vi "display_3s_stim_3s_ISI_9s_probes_trigger.vi"() -> ()   [LabVIEW 2019]
uses:
  <vilib>/Analysis/Matrix/Datatypes/RealMatrix.ctl
  <vilib>/Utility/file.llb/Write Delimited Spreadsheet (DBL).vi
  <vilib>/Analysis/Matrix/NI_Matrix.lvlib
panel:
  out "Num trials":u32=204
  out "ISI Time":dbl
  out "Stim TS":dbl
  out "Output":dbl[][](array[numeric])
  out "Output frame":T1
  out "Array temp1":T1
  out "Elapsed Time":dbl
  out "Display":bool=TRUE
  out "Trial":u32=1
  out "reward":dbl[](array[numeric])
  out "stim_id":dbl[](array[numeric])
  out "stim_loaded":dbl
  out "Timings":dbl[](array[numeric])
  out "Stimuli Loaded?":bool
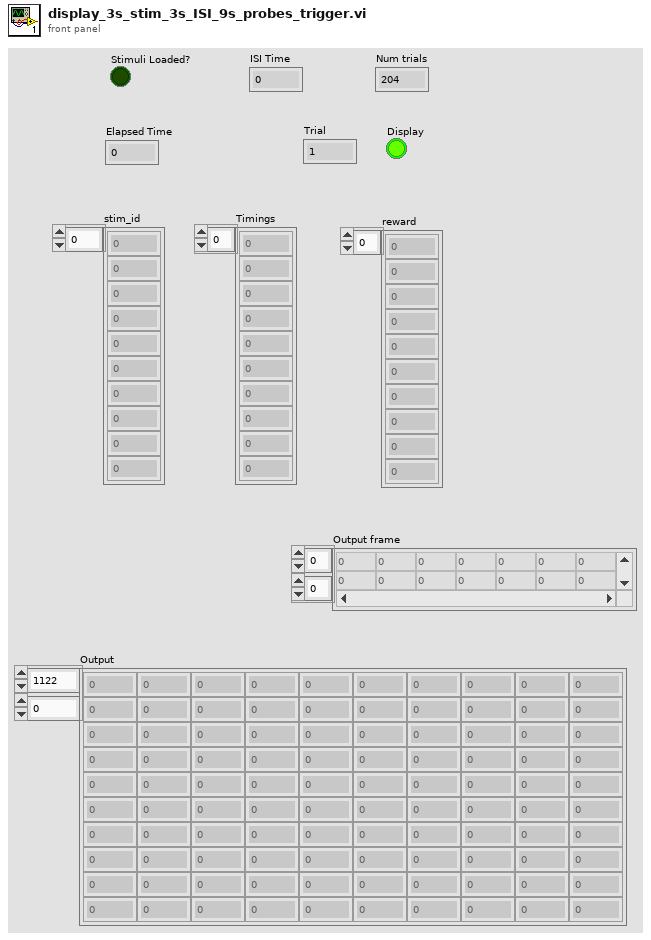
[diagram p1: front panel]
types:
  T1 = typedef "NI_Matrix.lvlib/RealMatrix.ctl" = dbl[][]
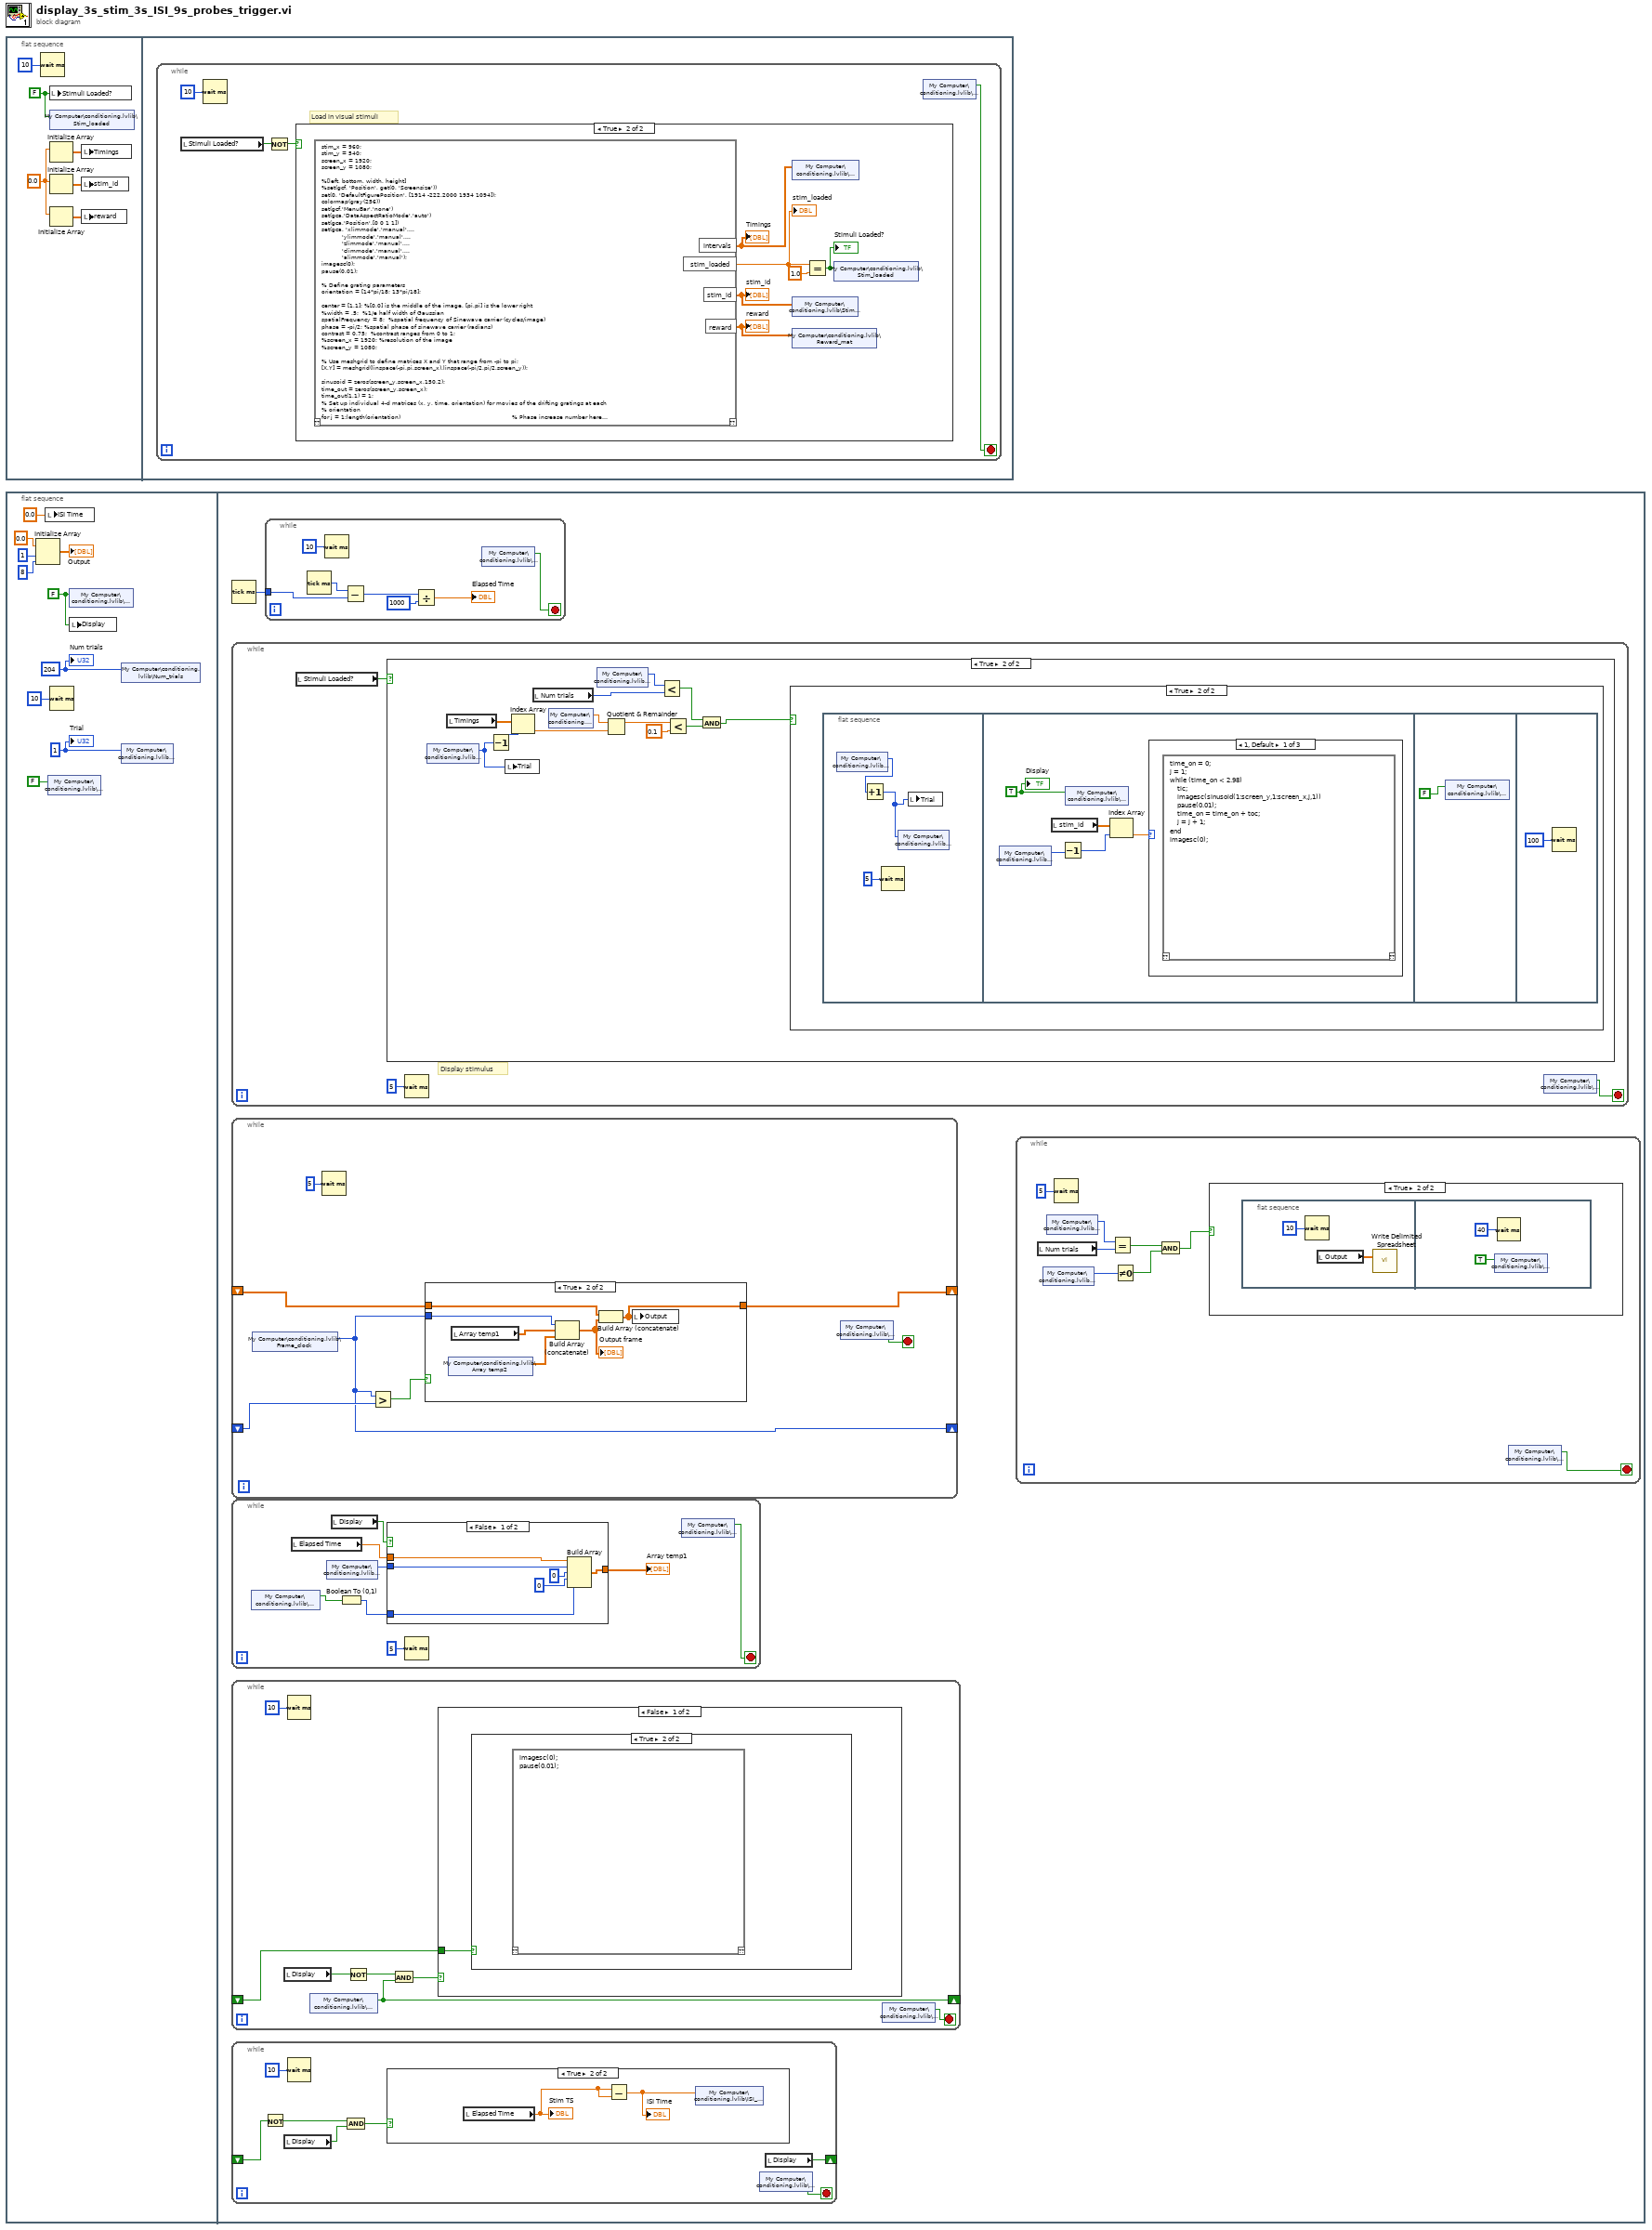
[diagram p0: block diagram]
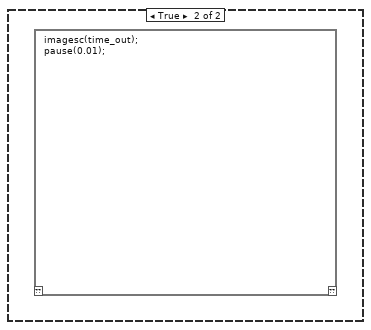
[diagram p5: hidden frame]
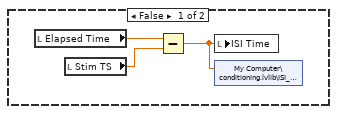
[diagram p6: hidden frame]
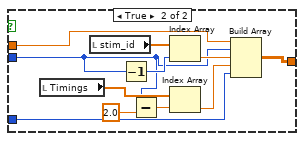
[diagram p7: hidden frame]
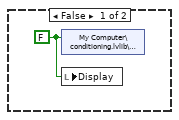
[diagram p10: hidden frame]
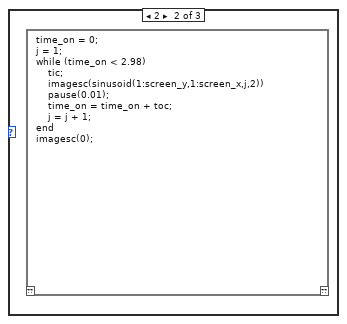
[diagram p11: hidden frame]
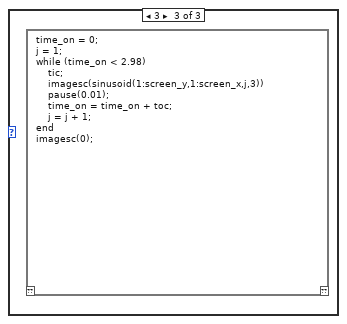
[diagram p12: hidden frame]
diagram:
  n1 = flat-sequence {
    frame #0 {
      w3 = 0.0 ("element")
      w1 = FALSE ("Stimuli Loaded?")
      n2 = Wait (ms)(milliseconds to wait=u32 10) -> ()  [unwired: 1 out]
      n3 = local write "Stimuli Loaded?"(w1) -> ()
      n4 = shared-variable "My Computer\\conditioning.lvlib\\Stim_loaded"(w1) -> ()  [unwired: 1 in, 1 out]
      n5 = Initialize Array(w3) -> (w5:dbl[])  [unwired: 1 in]
      n6 = Initialize Array(w3) -> (w4:dbl[])  [unwired: 1 in]
      n7 = Initialize Array(w3) -> (w2:dbl[])  [unwired: 1 in]
      n8 = local write "Timings"(w5) -> ()
      n9 = local write "stim_id"(w4) -> ()
      n10 = local write "reward"(w2) -> ()
    }
    frame #1 {
      n11 = while {
        stop <- w9 stop-if-true
        # "Load in visual stimuli"
        n12 = local read "Stimuli Loaded?"() -> (w8:bool)
        n13 = Wait (ms)(milliseconds to wait=u32 10) -> ()  [unwired: 1 out]
        n14 = Not(x=w8) -> (.not. x?=w7:bool)
        n15 = case shown="True" w7 {
          frame False {
          }
          frame True {
            n16 = script code="stim_x = 960;\nstim_y = 540;\nscreen_x = 1920;\nscreen_y = 1080;\n\n%[left, bottom, width, height]\n%set(gcf, 'Position', get(0, 'Screensize'))\nset(0, 'DefaultFigurePosition', [1914 -222.2000 1934 1094]);\ncolormap(gray(256))\nset(gcf,'MenuBar','none')\nset(gca,'DataAspectRatioMode','auto')\nset(gca,'Position',[0 0 1 1])\nset(gca, 'xlimmode','manual',...\n           'ylimmode','manual',...\n           'zlimmode','manual',...\n           'climmode','manual',...\n           'alimmode','manual');\nimagesc(0);\npause(0.01);\n\n% Define grating parameters\norientation = [14*pi/18; 13*pi/18];\n\ncenter = [1,1]; %[0,0] is the middle of the image, [pi,pi] is the lower right\n%width = .5;  %1/e half width of Gaussian\nspatialFrequency = 8;  %spatial frequency of Sinewave carrier (cycles/image)\nphase = -pi/2; %spatial phase of sinewave carrier (radians)\ncontrast = 0.75;  %contrast ranges from 0 to 1;\n%screen_x = 1920; %resolution of the image  \n%screen_y = 1080;\n\n% Use meshgrid to define matrices X and Y that range from -pi to pi;\n[X,Y] = meshgrid(linspace(-pi,pi,screen_x),linspace(-pi/2,pi/2,screen_y));\n\nsinusoid = zeros(screen_y,screen_x,150,2);\ntime_out = zeros(screen_y,screen_x);\ntime_out(1,1) = 1;\n% Set up individual 4-d matrices (x, y, time, orientation) for movies of the drifting gratings at each\n% orientation\nfor j = 1:length(orientation)                                                            % Phase increase number here\n    ramp(1:screen_y,1:screen_x,j) = cos(orientation(j))*(X-center(1)) + sin(orientation(j))*(Y-center(2));     %  |\n    for i = 1:150 %Sets the number of frames to define gratings for                   V\n       sinusoid(1:screen_y,1:screen_x,i,j) = contrast*sin(spatialFrequency*ramp(1:screen_y,1:screen_x,j)-...\n           (phase+(2*pi*(i-1)*(-30)/360))); %Number before '/360' sets the phase increase\n    end\nend\n\n%intervals = [ones(1,41)*10 ones(1,41)*11 ones(1,41)*12 ones(1,41)*13 ones(1,40)*14];\nintervals = [];\nfor i = 1:20\n   intervals = [intervals ones(1,9)*3 9];\nend\nintervals = [intervals 3 3 3 3];\n%intervals = [ones(1,204)*3];\nstim_id = [ones(1,204)*1];\n%reward = [ones(1,87)*1 ones(1,15)*0 ones(1,87)*1 ones(1,15)*0];\nreward = [ones(1,204)*1];\n\n%rand_idx1 = randperm(204);\n%rand_idx2 = randperm(204);\n%intervals = intervals(rand_idx2);\n%stim_id = stim_id(rand_idx2);\n%reward = reward(rand_idx2);\n\nstim_loaded = 1;" ("Script Node")() -> ("stim_loaded"=w16:dbl, "intervals"=w11:dbl[], "stim_id"=w12:dbl[], "reward"=w14:dbl[])  [unwired: 1 in, 1 out]
            "stim_loaded" <- w16
            "Timings" <- w11
            "stim_id" <- w12
            "reward" <- w14
            n17 = shared-variable "My Computer\\conditioning.lvlib\\Timings"(w11) -> ()  [unwired: 1 in, 1 out]
            n18 = shared-variable "My Computer\\conditioning.lvlib\\Stim_ID"(w12) -> ()  [unwired: 1 in, 1 out]
            n19 = shared-variable "My Computer\\conditioning.lvlib\\Reward_mat"(w14) -> ()  [unwired: 1 in, 1 out]
            n20 = Equal?(x=w16, y=1.0) -> (x = y?=w13:bool)
            "Stimuli Loaded?" <- w13
            n21 = shared-variable "My Computer\\conditioning.lvlib\\Stim_loaded"(w13) -> ()  [unwired: 1 in, 1 out]
          }
        }
        n22 = shared-variable "My Computer\\conditioning.lvlib\\Stop"() -> (w9:bool)  [unwired: 1 in, 1 out]
      }
    }
  }
  n23 = flat-sequence {
    frame #0 {
      w18 = u32 204
      w24 = FALSE ("Display")
      w26 = u32 1 ("Trial")
      n24 = Initialize Array(0.0 ("element"), 1 ("dimension size"), 8 ("dimension size")) -> (→"Output":dbl[][])
      n25 = local write "ISI Time"(0.0 ("ISI Time")) -> ()
      n26 = shared-variable "My Computer\\conditioning.lvlib\\Stop"(FALSE ("Stop")) -> ()  [unwired: 1 in, 1 out]
      n27 = Wait (ms)(milliseconds to wait=u32 10) -> ()  [unwired: 1 out]
      n28 = shared-variable "My Computer\\conditioning.lvlib\\Display"(w24) -> ()  [unwired: 1 in, 1 out]
      n29 = local write "Display"(w24) -> ()
      n30 = shared-variable "My Computer\\conditioning.lvlib\\Num_trials"(w18) -> ()  [unwired: 1 in, 1 out]
      n31 = shared-variable "My Computer\\conditioning.lvlib\\Trial"(w26) -> ()  [unwired: 1 in, 1 out]
      "Trial" <- w26
      "Num trials" <- w18
    }
    frame #1 {
      n32 = Tick Count (ms)() -> (millisecond timer value=w27:u32)
      n33 = while {
        stop <- w107 stop-if-true
        # "Display stimulus"
        n34 = local read "Stimuli Loaded?"() -> (w106:bool)
        n35 = case shown="True" w106 {
          frame False {
          }
          frame True {
            n36 = shared-variable "My Computer\\conditioning.lvlib\\Trial"() -> (w109:u32)  [unwired: 1 in, 1 out]
            n37 = local read "Timings"() -> (w118:dbl[])
            n38 = Decrement(x=w109) -> (x-1=w111:u32)
            n39 = local write "Trial"(w109) -> ()
            n40 = Index Array(array=w118, index=w111) -> (element=w117:dbl)
            n41 = local read "Num trials"() -> (w114:u32)
            n42 = shared-variable "My Computer\\conditioning.lvlib\\ISI"() -> (w113:dbl)  [unwired: 1 in, 1 out]
            n43 = shared-variable "My Computer\\conditioning.lvlib\\Trial"() -> (w110:u32)  [unwired: 1 in, 1 out]
            n44 = Quotient & Remainder(x=w113, y=w117) -> (x-y*floor(x/y)=w120:dbl)  [unwired: 1 out]
            n45 = Less?(x=w110, y=w114) -> (x < y?=w116:bool)
            n46 = Less?(x=w120, y=0.1) -> (x < y?=w115:bool)
            n47 = And(x=w116, y=w115) -> (x .and. y?=w112:bool)
            n48 = case shown="True" w112 {
              frame False {
                w121 = FALSE ("Display")
                n49 = shared-variable "My Computer\\conditioning.lvlib\\Display"(w121) -> ()  [unwired: 1 in, 1 out]
                n50 = local write "Display"(w121) -> ()
              }
              frame True {
                n51 = flat-sequence {
                  frame #0 {
                    n52 = shared-variable "My Computer\\conditioning.lvlib\\Trial"() -> (w123:u32)  [unwired: 1 in, 1 out]
                    n53 = Increment(x=w123) -> (x+1=w122:u32)
                    n54 = Wait (ms)(milliseconds to wait=u32 5) -> ()  [unwired: 1 out]
                    n55 = shared-variable "My Computer\\conditioning.lvlib\\Trial"(w122) -> ()  [unwired: 1 in, 1 out]
                    n56 = local write "Trial"(w122) -> ()
                  }
                  frame #1 {
                    w128 = TRUE ("Boolean")
                    n57 = shared-variable "My Computer\\conditioning.lvlib\\Trial"() -> (w125:u32)  [unwired: 1 in, 1 out]
                    n58 = local read "stim_id"() -> (w129:dbl[])
                    n59 = Decrement(x=w125) -> (x-1=w126:u32)
                    n60 = shared-variable "My Computer\\conditioning.lvlib\\Display"(w128) -> ()  [unwired: 1 in, 1 out]
                    n61 = Index Array(array=w129, index=w126) -> (element=w127:dbl)
                    n62 = case shown="1, Default" w127 {
                      frame 1, Default {
                        n63 = script code="time_on = 0;\nj = 1;\nwhile (time_on < 2.98)\n    tic;\n    imagesc(sinusoid(1:screen_y,1:screen_x,j,1))\n    pause(0.01);\n    time_on = time_on + toc;\n    j = j + 1;\nend\nimagesc(0);"() -> ()  [unwired: 1 in, 1 out]
                      }
                      frame 2 {
                        n64 = script code="time_on = 0;\nj = 1;\nwhile (time_on < 2.98)\n    tic;\n    imagesc(sinusoid(1:screen_y,1:screen_x,j,2))\n    pause(0.01);\n    time_on = time_on + toc;\n    j = j + 1;\nend\nimagesc(0);"() -> ()  [unwired: 1 in, 1 out]
                      }
                      frame 3 {
                        n65 = script code="time_on = 0;\nj = 1;\nwhile (time_on < 2.98)\n    tic;\n    imagesc(sinusoid(1:screen_y,1:screen_x,j,3))\n    pause(0.01);\n    time_on = time_on + toc;\n    j = j + 1;\nend\nimagesc(0);"() -> ()  [unwired: 1 in, 1 out]
                      }
                    }
                    "Display" <- w128
                  }
                  frame #2 {
                    n66 = shared-variable "My Computer\\conditioning.lvlib\\Display"(FALSE ("Display")) -> ()  [unwired: 1 in, 1 out]
                  }
                  frame #3 {
                    n67 = Wait (ms)(milliseconds to wait=u32 100) -> ()  [unwired: 1 out]
                  }
                }
              }
            }
          }
        }
        n68 = Wait (ms)(milliseconds to wait=u32 5) -> ()  [unwired: 1 out]
        n69 = shared-variable "My Computer\\conditioning.lvlib\\Stop"() -> (w107:bool)  [unwired: 1 in, 1 out]
      }
      n70 = while {
        shift-right: [w96] -> _
        shift-left: _ -> [w97]
        shift-right: [w93] -> _
        shift-left: _ -> [w95]
        stop <- w98 stop-if-true
        n71 = shared-variable "My Computer\\conditioning.lvlib\\Frame_clock"() -> (w93:u32)  [unwired: 1 in, 1 out]
        n72 = Wait (ms)(milliseconds to wait=u32 5) -> ()  [unwired: 1 out]
        n73 = Greater?(x=w93, y=w95) -> (0:w94:bool)
        n74 = case shown="True" w94 {
          tunnel: w97 -> [w99 w105]
          tunnel: [w99 w104] -> w96
          tunnel: w93 -> [_ w100]
          frame False {
          }
          frame True {
            n75 = shared-variable "My Computer\\conditioning.lvlib\\Array temp2"() -> (w102:dbl[][])  [unwired: 1 in, 1 out]
            n76 = local read "Array temp1"() -> (w103:T1)
            n77 = Build Array (concatenate)(w100, w103, w102) -> (w101:T1)
            "Output frame" <- w101
            n78 = Build Array (concatenate) ("Build Matrix")(w105, w101) -> (w104:T1)
            n79 = local write "Output"(w104) -> ()
          }
        }
        n80 = shared-variable "My Computer\\conditioning.lvlib\\Stop"() -> (w98:bool)  [unwired: 1 in, 1 out]
      }
      n81 = while {
        stop <- w62 stop-if-true
        n82 = shared-variable "My Computer\\conditioning.lvlib\\Timeout"() -> (w61:bool)  [unwired: 1 in, 1 out]
        n83 = local read "Elapsed Time"() -> (w66:dbl)
        n84 = shared-variable "My Computer\\conditioning.lvlib\\Trial"() -> (w64:u32)  [unwired: 1 in, 1 out]
        n85 = local read "Display"() -> (w63:bool)
        n86 = Boolean To (0,1)(Boolean=w61) -> (0, 1=w60:i16)
        n87 = case shown="False" w63 {
          tunnel: w64 -> [w72 w75]
          tunnel: w66 -> [w73 w82]
          tunnel: [w71 w83] -> w65
          tunnel: w60 -> [w68 w77]
          frame False {
            n88 = Build Array(w73, w72, u32 0 ("milliseconds to wait"), 0, w68) -> (w71:T1)
          }
          frame True {
            n89 = local read "Timings"() -> (w80:dbl[])
            n90 = local read "stim_id"() -> (w84:dbl[])
            n91 = Decrement(x=w75) -> (x-1=w79:u32)
            n92 = Subtract(x=w75, y=2.0) -> (x-y=w74:dbl)
            n93 = Index Array(array=w84, index=w79) -> (element=w81:dbl)
            n94 = Index Array(array=w80, index=w74) -> (element=w78:dbl)
            n95 = Build Array(w82, w75, w81, w78, w77) -> (w83:T1)
          }
        }
        "Array temp1" <- w65
        n96 = Wait (ms)(milliseconds to wait=u32 5) -> ()  [unwired: 1 out]
        n97 = shared-variable "My Computer\\conditioning.lvlib\\Stop"() -> (w62:bool)  [unwired: 1 in, 1 out]
      }
      n98 = while {
        shift-right: [w41] -> _
        shift-left: _ -> [w40]
        stop <- w46 stop-if-true
        n99 = local read "Display"() -> (w43:bool)
        n100 = Wait (ms)(milliseconds to wait=u32 10) -> ()  [unwired: 1 out]
        n101 = shared-variable "My Computer\\conditioning.lvlib\\Timeout"() -> (w41:bool)  [unwired: 1 in, 1 out]
        n102 = Not(x=w43) -> (.not. x?=w44:bool)
        n103 = And(x=w44, y=w41) -> (x .and. y?=w42:bool)
        n104 = case shown="False" w42 {
          tunnel: w40 -> [w47 _]
          frame False {
            n105 = case shown="True" w47 {
              frame False {
              }
              frame True {
                n106 = script code="imagesc(0);\npause(0.01);"() -> ()  [unwired: 1 in, 1 out]
              }
            }
          }
          frame True {
            n107 = script code="imagesc(time_out);\npause(0.01);"() -> ()  [unwired: 1 in, 1 out]
          }
        }
        n108 = shared-variable "My Computer\\conditioning.lvlib\\Stop"() -> (w46:bool)  [unwired: 1 in, 1 out]
      }
      n109 = while {
        shift-right: [w52] -> _
        shift-left: _ -> [w51]
        stop <- w54 stop-if-true
        n110 = Not(x=w51) -> (.not. x?=w50:bool)
        n111 = local read "Display"() -> (w49:bool)
        n112 = Wait (ms)(milliseconds to wait=u32 10) -> ()  [unwired: 1 out]
        n113 = And(x=w50, y=w49) -> (x .and. y?=w48:bool)
        n114 = case shown="True" w48 {
          frame False {
            n115 = local read "Elapsed Time"() -> (w55:dbl)
            n116 = local read "Stim TS"() -> (w57:dbl)
            n117 = Subtract(x=w55, y=w57) -> (x-y=w56:dbl)
            n118 = local write "ISI Time"(w56) -> ()
            n119 = shared-variable "My Computer\\conditioning.lvlib\\ISI_Time"(w56) -> ()  [unwired: 1 in, 1 out]
          }
          frame True {
            n120 = local read "Elapsed Time"() -> (w58:dbl)
            "Stim TS" <- w58
            n121 = Subtract(x=w58, y=w58) -> (x-y=w59:dbl)
            "ISI Time" <- w59
            n122 = shared-variable "My Computer\\conditioning.lvlib\\ISI_Time"(w59) -> ()  [unwired: 1 in, 1 out]
          }
        }
        n123 = shared-variable "My Computer\\conditioning.lvlib\\Stop"() -> (w54:bool)  [unwired: 1 in, 1 out]
        n124 = local read "Display"() -> (w52:bool)
      }
      n125 = while {
        tunnel: w27 -> [w88]
        stop <- w85 stop-if-true
        n126 = Tick Count (ms)() -> (millisecond timer value=w89:u32)
        n127 = Wait (ms)(milliseconds to wait=u32 10) -> ()  [unwired: 1 out]
        n128 = Subtract(x=w89, y=w88) -> (x-y=w86:u32)
        n129 = Divide(x=w86, y=u32 1000) -> (x/y=→"Elapsed Time":dbl)
        n130 = shared-variable "My Computer\\conditioning.lvlib\\Stop"() -> (w85:bool)  [unwired: 1 in, 1 out]
      }
      n131 = while {
        stop <- w28 stop-if-true
        n132 = local read "Num trials"() -> (w32:u32)
        n133 = shared-variable "My Computer\\conditioning.lvlib\\Trial"() -> (w35:u32)  [unwired: 1 in, 1 out]
        n134 = shared-variable "My Computer\\conditioning.lvlib\\Trial"() -> (w31:u32)  [unwired: 1 in, 1 out]
        n135 = Wait (ms)(milliseconds to wait=u32 5) -> ()  [unwired: 1 out]
        n136 = Equal?(x=w31, y=w32) -> (x = y?=w33:bool)
        n137 = Not Equal To 0?(x=w35) -> (x != 0?=w34:bool)
        n138 = And(x=w33, y=w34) -> (x .and. y?=w29:bool)
        n139 = case shown="True" w29 {
          frame False {
          }
          frame True {
            n140 = flat-sequence {
              frame #0 {
                n141 = Wait (ms)(milliseconds to wait=u32 10) -> ()  [unwired: 1 out]
                n142 = local read "Output"() -> (w37:dbl[][])
                n143 = call-poly <vilib>:"Write Delimited Spreadsheet.vi"("2D data"=w37) -> ()  [unwired: 13 in, 2 out]
              }
              frame #1 {
                n144 = shared-variable "My Computer\\conditioning.lvlib\\Stop"(TRUE) -> ()  [unwired: 1 in, 1 out]
                n145 = Wait (ms)(milliseconds to wait=u32 40) -> ()  [unwired: 1 out]
              }
            }
          }
        }
        n146 = shared-variable "My Computer\\conditioning.lvlib\\Stop"() -> (w28:bool)  [unwired: 1 in, 1 out]
      }
    }
  }
